vi "MacroEditor.vi"(2 "System":u16(ring) items=["Cusp", "Positron", "Musashi"], 3 "Save/Open Path":path=path "C:/CuspControl/Cusp/1_Macros/Antiprotons/Reservoir/Test1/scoop.mac", 4 "Sub-vi'd (open)":bool=TRUE) -> (1 "Saved at least once":bool=TRUE)   [LabVIEW 2018]
uses:
  MacroEditor Files/Instructions.ctl
  Executor Files/RT/Instruction.ctl
  Executor Files/VariableScan_Cluster.ctl
  MacroEditor Files/MacroSaveCluster.ctl
panel:
  in  "Tab Control":enum32{"Main", "Stored", "Basher"}(tab)
  in  "Instructions":T1=[{"Duration"=0.1, "Comment"="wait", "Steps"=1, "Edit Potential"=FALSE, "Output Bits"=[FALSE, FALSE, FALSE, FALSE, FALSE, FALSE, FALSE, FALSE, FALSE, FALSE, FALSE, FALSE, FALSE, FALSE, FALSE, FALSE, FALSE, FALSE, FALSE, FALSE, FALSE, FALSE, FALSE, FALSE, FALSE, FALSE, FALSE, FALSE, FALSE, FALSE, FALSE, FALSE, FALSE, FALSE, FALSE, FALSE, FALSE, FALSE], "Macro Path"=path "", "Potentials"=[-100.0, 0.0, -14.0, 0.0, 0.0, 0.0, -100.0, 0.0, 0.0, 0.0, 0.0, 0.0, 0.0, 0.0, 0.0, 0.0], "Inherit?"=FALSE}, {"Duration"=0.1, "Comment"="pbar to u8u9\nrw off", "Steps"=100, "Edit Potential"=FALSE, "Output Bits"=[FALSE, FALSE, FALSE, FALSE, FALSE, FALSE, FALSE, FALSE, FALSE, FALSE, FALSE, FALSE, FALSE, FALSE, FALSE, FALSE, FALSE, FALSE, FALSE, FALSE, FALSE, FALSE, FALSE, FALSE, FALSE, FALSE, FALSE, FALSE, FALSE, FALSE, FALSE, FALSE, FALSE, FALSE, FALSE, FALSE, FALSE, FALSE], "Macro Path"=path "", "Potentials"=[-100.0, 0.0, 0.0, 0.0, 20.0, 20.0, -100.0, 0.0, 0.0, 0.0, 0.0, 0.0, 0.0, 0.0, 0.0, 0.0], "Inherit?"=FALSE}, {"Duration"=0.1, "Comment"="match level", "Steps"=100, "Edit Potential"=FALSE, "Output Bits"=[FALSE, FALSE, FALSE, FALSE, FALSE, FALSE, FALSE, FALSE, FALSE, FALSE, FALSE, FALSE, FALSE, FALSE, FALSE, FALSE, FALSE, FALSE, FALSE, FALSE, FALSE, FALSE, FALSE, FALSE, FALSE, FALSE, FALSE, FALSE, FALSE, FALSE, FALSE, FALSE, FALSE, FALSE, FALSE, FALSE, FALSE, FALSE], "Macro Path"=path "", "Potentials"=[-100.0, 0.0, 0.0, 0.0, 1.93, 1.93, -100.0, 0.0, 0.0, 0.0, 0.0, 0.0, 0.0, 0.0, 0.0, 0.0], "Inherit?"=FALSE}, {"Duration"=0.1, "Comment"="scoop", "Steps"=100, "Edit Potential"=FALSE, "Output Bits"=[FALSE, FALSE, FALSE, FALSE, FALSE, FALSE, FALSE, FALSE, FALSE, FALSE, FALSE, FALSE, FALSE, FALSE, FALSE, FALSE, FALSE, FALSE, FALSE, FALSE, FALSE, FALSE, FALSE, FALSE, FALSE, FALSE, FALSE, FALSE, FALSE, FALSE, FALSE, FALSE, FALSE, FALSE, FALSE, FALSE, FALSE, FALSE], "Macro Path"=path "", "Potentials"=[-100.0, 80.0, -50.0, 0.0, 1.93, 1.93, -100.0, 0.0, 0.0, 0.0, 0.0, 0.0, 0.0, 0.0, 0.0, 0.0], "Inherit?"=FALSE}, {"Duration"=0.1, "Comment"="move\n12: u13 relay", "Steps"=100, "Edit Potential"=FALSE, "Output Bits"=[FALSE, FALSE, FALSE, FALSE, FALSE, FALSE, FALSE, FALSE, FALSE, FALSE, FALSE, FALSE, TRUE, FALSE, FALSE, FALSE, FALSE, FALSE, FALSE, FALSE, FALSE, FALSE, FALSE, FALSE, FALSE, FALSE, FALSE, FALSE, FALSE, FALSE, FALSE, FALSE, FALSE, FALSE, FALSE, FALSE, FALSE, FALSE], "Macro Path"=path "", "Potentials"=[-100.0, 70.0, -110.0, 0.0, 20.0, 20.0, -100.0, 0.0, 0.0, 0.0, 0.0, 0.0, 0.0, 0.0, 0.0, 0.0], "Inherit?"=FALSE}, {"Duration"=0.1, "Comment"="move\n", "Steps"=100, "Edit Potential"=FALSE, "Output Bits"=[FALSE, FALSE, FALSE, FALSE, FALSE, FALSE, FALSE, FALSE, FALSE, FALSE, FALSE, FALSE, TRUE, FALSE, FALSE, FALSE, FALSE, FALSE, FALSE, FALSE, FALSE, FALSE, FALSE, FALSE, FALSE, FALSE, FALSE, FALSE, FALSE, FALSE, FALSE, FALSE, FALSE, FALSE, FALSE, FALSE, FALSE, FALSE], "Macro Path"=path "", "Potentials"=[-100.0, -95.0, -110.0, 0.0, 20.0, 20.0, -100.0, 0.0, 0.0, 0.0, 0.0, 0.0, 0.0, 0.0, 0.0, 0.0], "Inherit?"=FALSE}, {"Duration"=0.005, "Comment"="01: ekick", "Steps"=1, "Edit Potential"=FALSE, "Output Bits"=[FALSE, TRUE, FALSE, FALSE, FALSE, FALSE, FALSE, FALSE, FALSE, FALSE, FALSE, FALSE, TRUE, FALSE, FALSE, FALSE, FALSE, FALSE, FALSE, FALSE, FALSE, FALSE, FALSE, FALSE, FALSE, FALSE, FALSE, FALSE, FALSE, FALSE, FALSE, FALSE, FALSE, FALSE, FALSE, FALSE, FALSE, FALSE], "Macro Path"=path "", "Potentials"=[-100.0, -95.0, -110.0, 0.0, 20.0, 20.0, -100.0, 0.0, 0.0, 0.0, 0.0, 0.0, 0.0, 0.0, 0.0, 0.0], "Inherit?"=TRUE}, {"Duration"=0.005, "Comment"="dump\n00: daq trig\n23: hodo trig", "Steps"=1, "Edit Potential"=FALSE, "Output Bits"=[TRUE, FALSE, FALSE, FALSE, FALSE, FALSE, FALSE, FALSE, FALSE, FALSE, FALSE, FALSE, TRUE, FALSE, FALSE, FALSE, FALSE, FALSE, FALSE, FALSE, FALSE, FALSE, FALSE, TRUE, FALSE, FALSE, FALSE, FALSE, FALSE, FALSE, FALSE, FALSE, FALSE, FALSE, FALSE, FALSE, FALSE, FALSE], "Macro Path"=path "", "Potentials"=[-100.0, -130.0, -110.0, 0.0, 20.0, 20.0, -100.0, 0.0, 0.0, 0.0, 0.0, 0.0, 0.0, 0.0, 0.0, 0.0], "Inherit?"=FALSE}, {"Duration"=0.01, "Comment"="recover", "Steps"=100, "Edit Potential"=FALSE, "Output Bits"=[FALSE, FALSE, FALSE, FALSE, FALSE, FALSE, FALSE, FALSE, FALSE, FALSE, FALSE, FALSE, FALSE, FALSE, FALSE, FALSE, FALSE, FALSE, FALSE, FALSE, FALSE, FALSE, FALSE, FALSE, FALSE, FALSE, FALSE, FALSE, FALSE, FALSE, FALSE, FALSE, FALSE, FALSE, FALSE, FALSE, FALSE, FALSE], "Macro Path"=path "", "Potentials"=[-100.0, 0.0, -14.0, 0.0, 20.0, 20.0, -100.0, 0.0, 0.0, 0.0, 0.0, 0.0, 0.0, 0.0, 0.0, 0.0], "Inherit?"=FALSE}, {"Duration"=0.1, "Comment"="back to rw well", "Steps"=100, "Edit Potential"=FALSE, "Output Bits"=[FALSE, FALSE, FALSE, FALSE, FALSE, FALSE, FALSE, FALSE, FALSE, FALSE, FALSE, FALSE, FALSE, FALSE, FALSE, FALSE, FALSE, FALSE, FALSE, FALSE, FALSE, FALSE, FALSE, FALSE, FALSE, FALSE, FALSE, FALSE, FALSE, FALSE, FALSE, FALSE, FALSE, FALSE, FALSE, FALSE, FALSE, FALSE], "Macro Path"=path "", "Potentials"=[-100.0, 0.0, -14.0, 0.0, 0.0, 0.0, -100.0, 0.0, 0.0, 0.0, 0.0, 0.0, 0.0, 0.0, 0.0, 0.0], "Inherit?"=FALSE}] {"Steps" min=1 max=100000 step=1; "Duration" min=0.001 step=0.001 format="%_6p"}
  in  "stop":bool
  in  "Save":bool
  in  "Open":bool
  in  "New":bool
  in  "Macro Description":string="start and end in pbar rw well\ne+ stay in u7 = -100 V"
  in  "Copy Inst.":bool
  out "Changes":bool[][](array[boolean])=[[TRUE, TRUE], [FALSE, TRUE], [FALSE, TRUE], [FALSE, TRUE], [TRUE, TRUE], [FALSE, TRUE], [TRUE, FALSE], [TRUE, TRUE], [TRUE, TRUE], [FALSE, TRUE]]
  out "message":string="Input Bit Assignments\n-------------------------\n01 pbar sync\n02 e+ sync\n\nOutput Bit Assignments\n-------------------------\n00 DAQ trigger\n01 HV pulser(s) trigger\n02 \n03 MCP select\n04 MCP in\n05 MCP out\n06 e- source select\n07 e- source insert\n08 e- source remove\n09 pulsed coil enable\n10 Brescia trigger\n11 Relays - u10\n12 AC bypass relay - u13\n13 Entrance GV open\n14 Entrance GV close\n15 bk4054b gate - u5\n16 bk4054b gate - u10\n17 Higaki B-C fire\n18 Higaki A fire\n19 Tajima fire\n20 Tanaka fire\n21 Exit GV open\n22 Exit GV close\n23 BGO gate\n24 bk4054b gate - u4"
  out "# Instructions":i32=10
  out "Total time (s)":dbl=0.738 format="%_4p"
  in  "Analog buffer (2 ms)":dbl=0.002 format="%#_3p"
  in  "Path tag":string="t"
  in  "Variable Cluster":T3={"Values"=[2.78, 1.795, 0.81, -0.17499999999999982, -1.16], "Action"=1, "Inst."=2, "# Elements"=5, "Next Element"=0, "First Val"=2.78, "Final Val"=-1.16, "Update Array"=FALSE, "Description"="", "Variable Type"=1, "Scan Now"=FALSE, "# Act/Inst."=2, "Electrodes_range"=[], "Parameter Name"="RW&f_start (Hz)", "# Passes"=1} {"Variable Type" items=["Duration (s)", "Voltage (V)", "Parameter", "Repetitions"]; "Final Val" format="%_6p"; "First Val" format="%_6p"; "Values" format="%_6p"}
  out "Edit #":i32=-1
  # "0        2       4       6        8      10     12     14     16     18      20    22     24     26     28     30     32     34     36"
  # "Digital and Analog 'Changes' is only updated when you Save"
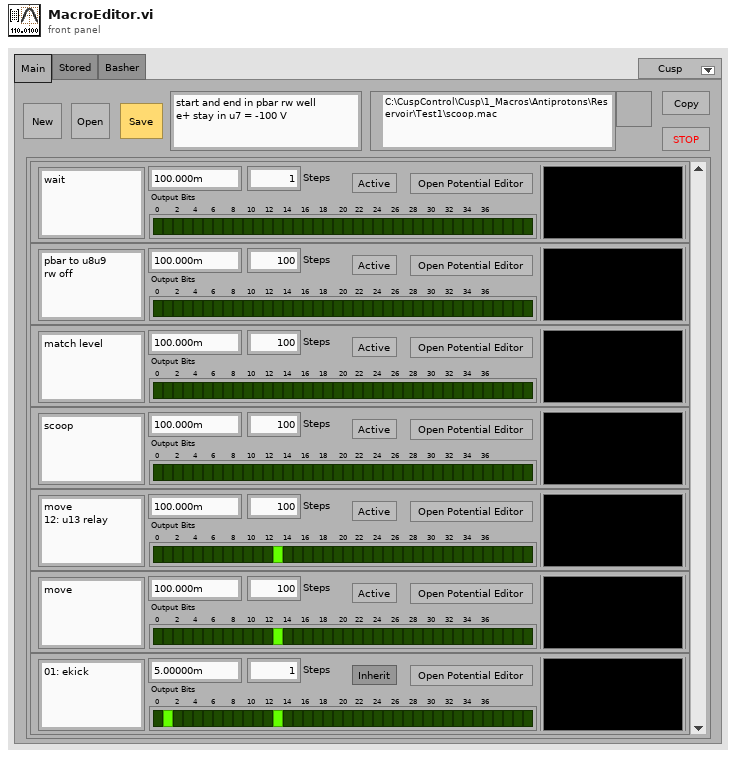
[diagram p1: front panel]
types:
  T1 = typedef "Instructions.ctl" = T2[]
  T2 = typedef "Instruction.ctl" = cluster{"Duration":dbl, "Comment":string, "Steps":i32, "Edit Potential":bool, "Output Bits":bool[], "Macro Path":path, "Potentials":dbl[], "Inherit?":bool}
  T3 = typedef "VariableScan_Cluster.ctl" = cluster{"Values":dbl[], "Action":i32, "Inst.":i32, "# Elements":i32, "Next Element":i32, "First Val":dbl, "Final Val":dbl, "Update Array":bool, "Description":string, "Variable Type":u16, "Scan Now":bool, "# Act/Inst.":i32, "Electrodes_range":i32[], "Parameter Name":string, "# Passes":i32}
  T4 = typedef "MacroSaveCluster.ctl" = cluster{"Instructions":T1, "Changes":bool[][], "Macro Description":string, "Total Time (s)":dbl, "Samples per sec":dbl}
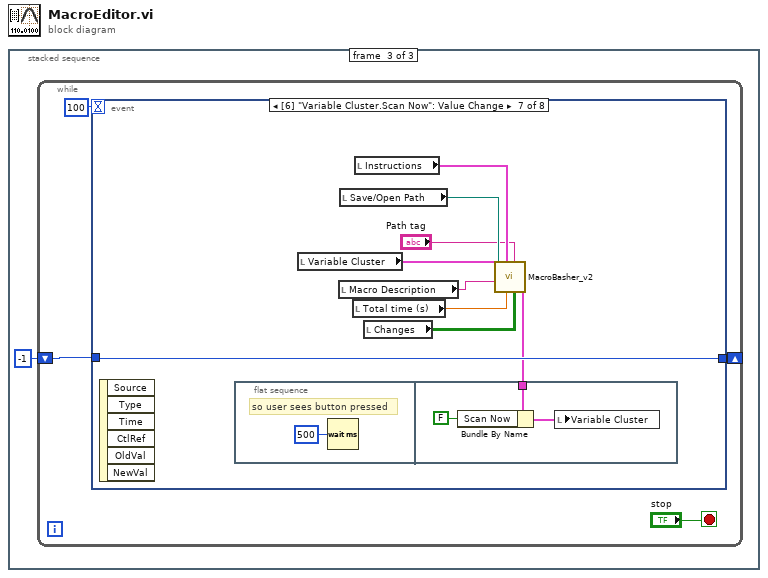
[diagram p0: block diagram]
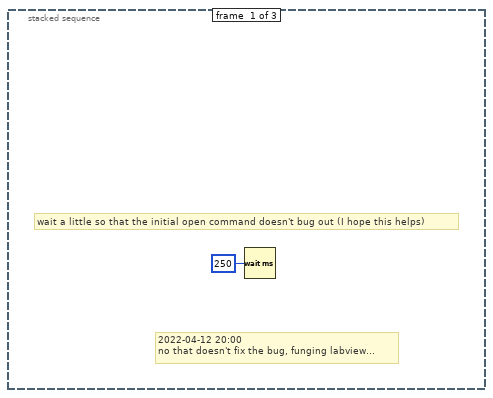
[diagram p2: hidden frame]
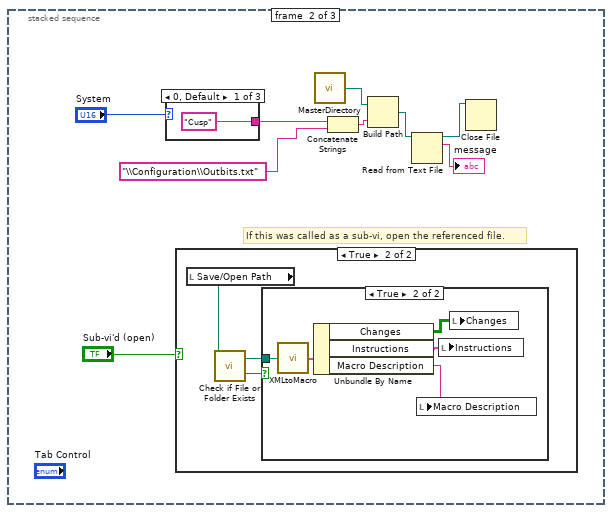
[diagram p3: hidden frame]
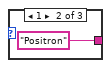
[diagram p4: hidden frame]
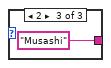
[diagram p5: hidden frame]
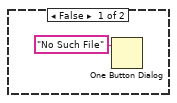
[diagram p7: hidden frame]
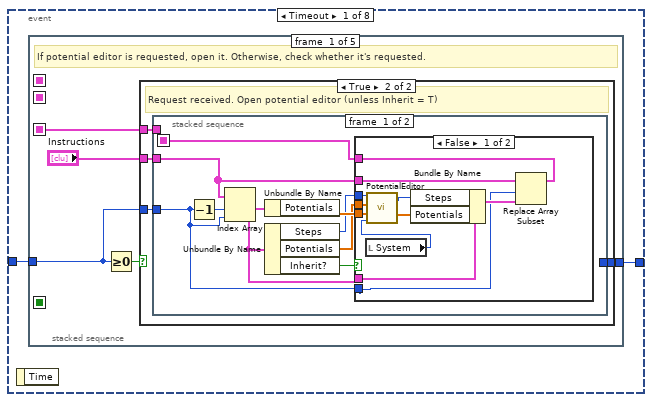
[diagram p8: hidden frame]
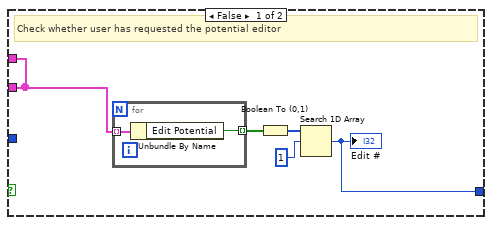
[diagram p9: hidden frame]
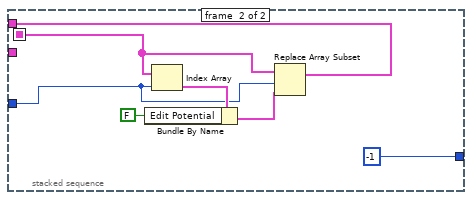
[diagram p11: hidden frame]
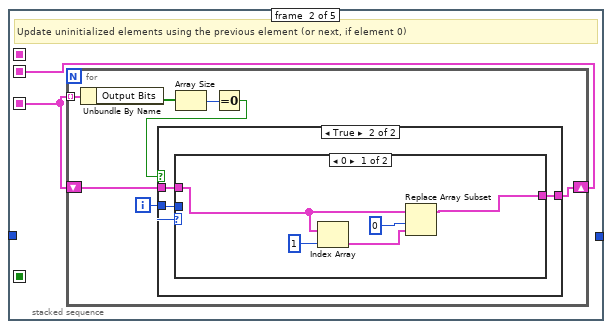
[diagram p12: hidden frame]
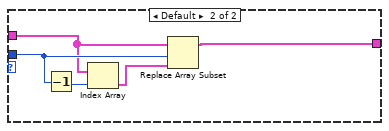
[diagram p14: hidden frame]
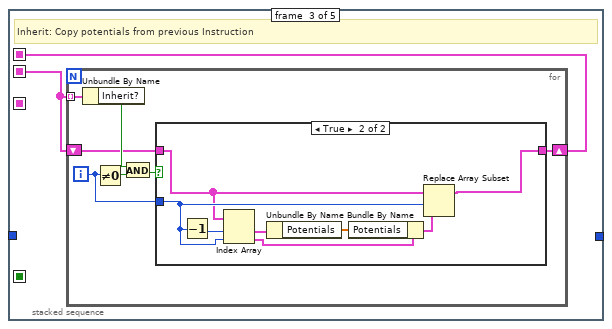
[diagram p15: hidden frame]
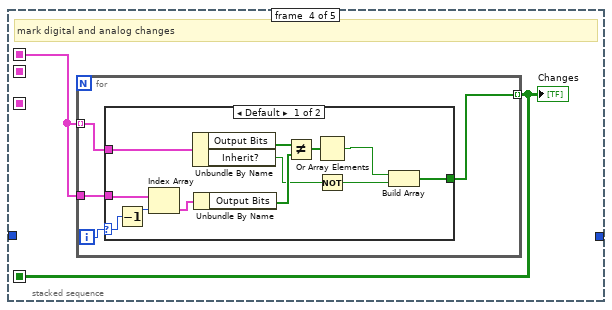
[diagram p17: hidden frame]
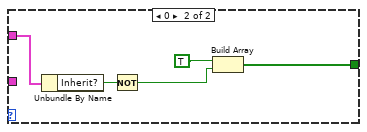
[diagram p18: hidden frame]
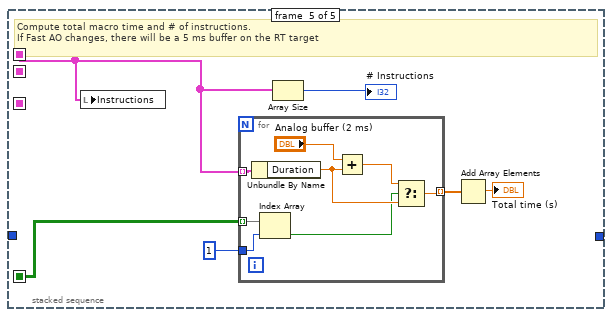
[diagram p19: hidden frame]
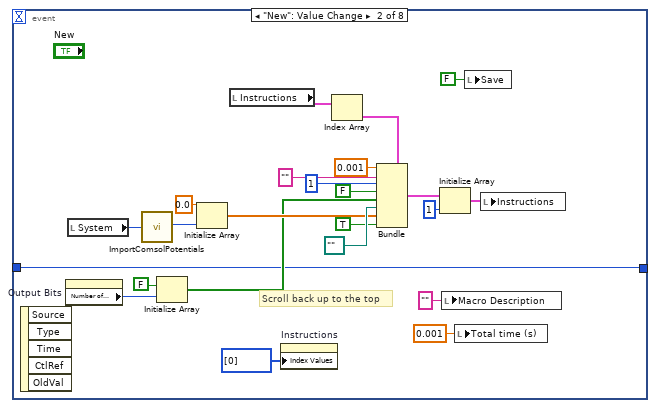
[diagram p20: hidden frame]
diagram:
  n1 = stacked-sequence {
    frame #0 {
      # "2022-04-12 20:00\nno that doesn't fix the bug, funging labview..."
      # "wait a little so that the initial open command doesn't bug out (I hope this helps)"
      n2 = Wait (ms)(milliseconds to wait=u32 250) -> ()  [unwired: 1 out]
    }
    frame #1 {
      # "If this was called as a sub-vi, open the referenced file."
      n3 = case shown="0, Default" "System" {
        tunnel: ["Cusp" ("string") "Positron" ("string") "Musashi" ("string")] -> w9
        frame 0, Default {
        }
        frame 1 {
        }
        frame 2 {
        }
      }
      n4 = case shown="True" "Sub-vi'd (open)" {
        frame False {
        }
        frame True {
          n5 = local read "Save/Open Path"() -> (w14:path)
          n6 = call <vilib>:"Check if File or Folder Exists.vi"("path"=w14) -> ("file or folder exists?"=w16:bool, "dup path"=w15:path)  [unwired: 8 in, 1 out]
          n7 = case shown="True" w16 {
            tunnel: w15 -> [_ w22]
            frame False {
              n8 = One Button Dialog(message="No Such File") -> ()  [unwired: 1 in, 1 out]
            }
            frame True {
              n9 = call "XMLtoMacro.vi"("XML File Path"=w22) -> ("MacroSaveCluster"=w21:T4)
              n10 = Unbundle By Name(w21) -> ("Changes"=w19:bool[][], "Instructions"=w18:T1, "Macro Description"=w20:string)
              n11 = local write "Macro Description"(w20) -> ()
              n12 = local write "Instructions"(w18) -> ()
              n13 = local write "Changes"(w19) -> ()
            }
          }
        }
      }
      n14 = call "MasterDirectory.vi"() -> ("Master Directory"=w5:path)
      n15 = Concatenate Strings(w9, "\\Configuration\\Outbits.txt" ("string")) -> (w4:string)
      n16 = Build Path(base path=w5, name or relative path=w4) -> (appended path=w3:path)
      n17 = Read from Text File(file (use dialog)=w3) -> (refnum out=w6:refnum<file>, text=→"message":string)  [unwired: 3 in, 2 out]
      n18 = Close File(refnum=w6) -> ()  [unwired: 1 in, 2 out]
    }
    frame #2 {
      n19 = while {
        shift-right: [w24] -> _
        shift-left: -1 ("Edit #") -> [w25]
        stop <- "stop" stop-if-true
        n20 = event shown="[6] \"Variable Cluster.Scan Now\": Value Change" {
          selector: _ -> [_ _ _ _ _ _ _ _]
          dyn-events: _ -> [_ _ _ _ _ _ _ _]
          timeout: 100 -> [_ _ _ _ _ _ _ _]
          tunnel: w25 -> [w29 w153 w176 w188 w199 w201 w213 w219]
          tunnel: [w28 w153 w176 w188 w199 w201 w213 w219] -> w24
          event Timeout {
            n21 = event-data() -> ()  [unwired: 1 in, 1 out]
            n22 = stacked-sequence {
              seq-local: [w32 _ _ _ _] -> [_ w76 _ _ _]
              seq-local: [_ w75 _ _ _] -> [_ _ w99 _ _]
              seq-local: [_ _ w98 _ _] -> [_ _ _ w117 w139]
              seq-local: [_ _ _ w116 _] -> [_ _ _ _ w140]
              tunnel: w29 -> [w31 _ _ _ _]
              tunnel: [w30 _ _ _ _] -> w28
              frame #0 {
                # "If potential editor is requested, open it. Otherwise, check whether it's requested."
                n23 = Greater Or Equal To 0?(x=w31) -> (x >= 0?=w34:bool)
                n24 = case shown="True" w34 {
                  tunnel: w31 -> [_ w45]
                  tunnel: "Instructions" -> [w36 w44]
                  tunnel: [w36 w43] -> w32
                  tunnel: [w35 w42] -> w30
                  frame False {
                    # "Check whether user has requested the potential editor"
                    n25 = for {
                      tunnel: w36 -> [w41] mode=indexing
                      tunnel: [w40] -> w37 mode=indexing
                      n26 = Unbundle By Name(w41) -> ("Edit Potential"=w40:bool)
                    }
                    n27 = Boolean To (0,1)(Boolean=w37) -> (0, 1=w39:i16[])
                    n28 = Search 1D Array(1D array=w39, element=1) -> (index of element=w35:i32)  [unwired: 1 in]
                    "Edit #" <- w35
                  }
                  frame True {
                    # "Request received. Open potential editor (unless Inherit = T)"
                    n29 = stacked-sequence {
                      seq-local: [w47 _] -> [_ w70]
                      tunnel: w45 -> [w46 w72]
                      tunnel: w44 -> [w48 _]
                      tunnel: [_ w69] -> w43
                      tunnel: [_ -1 ("Edit #")] -> w42
                      frame #0 {
                        n30 = Decrement(x=w46) -> (x-1=w55:i32)
                        n31 = Index Array(array=w48, index #1=w55, index #2=w46) -> (element #1=w54:T2, element #2=w50:T2)
                        n32 = Unbundle By Name(w54) -> ("Potentials"=w53:dbl[])
                        n33 = Unbundle By Name(w50) -> ("Steps"=w51:i32, "Potentials"=w52:dbl[], "Inherit?"=w49:bool)
                        n34 = case shown="False" w49 {
                          tunnel: w53 -> [w66 _]
                          tunnel: w52 -> [w65 _]
                          tunnel: w51 -> [w64 _]
                          tunnel: w50 -> [w63 _]
                          tunnel: w48 -> [w59 w67]
                          tunnel: [w57 w67] -> w47
                          tunnel: w46 -> [w56 _]
                          frame False {
                            n35 = local read "System"() -> (w58:u16)
                            n36 = call "PotentialEditor.vi"("System"=w58, "Previous Excitations in"=w66, "Requested"=w65, "Steps"=w64) -> ("Excitations Out"=w62:dbl[], "Steps Out"=w61:i32)
                            n37 = Bundle By Name(cluster=w63, "Steps"=w61, "Potentials"=w62) -> (w60:T2)
                            n38 = Replace Array Subset(array=w59, new element=w60, index=w56) -> (w57:T1)
                          }
                          frame True {
                          }
                        }
                      }
                      frame #1 {
                        n39 = Index Array(array=w70, index=w72) -> (element=w74:T2)
                        n40 = Bundle By Name(cluster=w74, "Edit Potential"=FALSE) -> (w71:T2)
                        n41 = Replace Array Subset(array=w70, new element=w71, index=w72) -> (w69:T1)
                      }
                    }
                  }
                }
              }
              frame #1 {
                # "Update uninitialized elements using the previous element (or next, if element 0)"
                n42 = for {
                  tunnel: w76 -> [w83] mode=indexing
                  shift-right: [w77] -> w75
                  shift-left: w76 -> [w78]
                  i -> [w80]
                  n43 = Unbundle By Name(w83) -> ("Output Bits"=w82:bool[])
                  n44 = Array Size(array=w82) -> (size(s)=w81:i32)
                  n45 = Equal To 0?(x=w81) -> (x = 0?=w79:bool)
                  n46 = case shown="True" w79 {
                    tunnel: w80 -> [_ w87]
                    tunnel: w78 -> [w84 w86]
                    tunnel: [w84 w85] -> w77
                    frame False {
                    }
                    frame True {
                      n47 = case shown="0" w87 {
                        tunnel: w87 -> [_ w96]
                        tunnel: w86 -> [w89 w94]
                        tunnel: [w88 w93] -> w85
                        frame 0 {
                          n48 = Index Array(array=w89, index=1) -> (element=w90:T2)
                          n49 = Replace Array Subset(array=w89, new element=w90, index=0) -> (w88:T1)
                        }
                        frame Default {
                          n50 = Decrement(x=w96) -> (x-1=w97:i32)
                          n51 = Index Array(array=w94, index=w97) -> (element=w95:T2)
                          n52 = Replace Array Subset(array=w94, new element=w95, index=w96) -> (w93:T1)
                        }
                      }
                    }
                  }
                }
              }
              frame #2 {
                # "Inherit: Copy potentials from previous Instruction"
                n53 = for {
                  tunnel: w99 -> [w106] mode=indexing
                  shift-right: [w100] -> w98
                  shift-left: w99 -> [w101]
                  i -> [w103]
                  n54 = Unbundle By Name(w106) -> ("Inherit?"=w104:bool)
                  n55 = Not Equal To 0?(x=w103) -> (x != 0?=w102:bool)
                  n56 = And(x=w104, y=w102) -> (x .and. y?=w105:bool)
                  n57 = case shown="True" w105 {
                    tunnel: w103 -> [_ w113]
                    tunnel: w101 -> [w107 w109]
                    tunnel: [w107 w108] -> w100
                    frame False {
                    }
                    frame True {
                      n58 = Decrement(x=w113) -> (x-1=w115:i32)
                      n59 = Index Array(array=w109, index #1=w115, index #2=w113) -> (element #1=w114:T2, element #2=w112:T2)
                      n60 = Unbundle By Name(w114) -> ("Potentials"=w111:dbl[])
                      n61 = Bundle By Name(cluster=w112, "Potentials"=w111) -> (w110:T2)
                      n62 = Replace Array Subset(array=w109, new element=w110, index=w113) -> (w108:T1)
                    }
                  }
                }
              }
              frame #3 {
                # "mark digital and analog changes"
                n63 = for {
                  tunnel: w117 -> [w120] mode=indexing
                  tunnel: [w118] -> w116 mode=indexing
                  tunnel: w117 -> [w119]
                  i -> [w121]
                  n64 = case shown="Default" w121 {
                    selector: w121 -> [w131 _]
                    tunnel: [w124 w137] -> w118
                    tunnel: w120 -> [w130 w136]
                    tunnel: w119 -> [w133 _]
                    frame Default {
                      n65 = Decrement(x=w131) -> (x-1=w132:i32)
                      n66 = Index Array(array=w133, index=w132) -> (element=w129:T2)
                      n67 = Unbundle By Name(w130) -> ("Output Bits"=w128:bool[], "Inherit?"=w123:bool)
                      n68 = Unbundle By Name(w129) -> ("Output Bits"=w127:bool[])
                      n69 = Not Equal?(x=w128, y=w127) -> (x != y?=w126:bool[])
                      n70 = Or Array Elements(Boolean array=w126) -> (logical OR=w125:bool)
                      n71 = Not(x=w123) -> (.not. x?=w122:bool)
                      n72 = Build Array(w125, w122) -> (w124:bool[])
                    }
                    frame 0 {
                      n73 = Unbundle By Name(w136) -> ("Inherit?"=w135:bool)
                      n74 = Not(x=w135) -> (.not. x?=w134:bool)
                      n75 = Build Array(TRUE, w134) -> (w137:bool[])
                    }
                  }
                }
                "Changes" <- w116
              }
              frame #4 {
                # "Compute total macro time and # of instructions.\nIf Fast AO changes, there will be a 5 ms buffer on the RT target"
                n76 = local write "Instructions"(w139) -> ()
                n77 = for {
                  tunnel: w139 -> [w152] mode=indexing
                  tunnel: [w150] -> w144 mode=indexing
                  tunnel: w140 -> [w147] mode=indexing
                  tunnel: 1 ("index") -> [w146]
                  n78 = Unbundle By Name(w152) -> ("Duration"=w148:dbl)
                  n79 = Index Array(array=w147, index=w146) -> (element=w145:bool)
                  n80 = Add(x="Analog buffer (2 ms)", y=w148) -> (x+y=w149:dbl)
                  n81 = Select(t=w149, s=w145, f=w148) -> (s? t:f=w150:dbl)
                }
                n82 = Array Size(array=w139) -> (size(s)=→"# Instructions":i32)
                n83 = Add Array Elements(numeric array=w144) -> (sum=→"Total time (s)":dbl)
              }
            }
          }
          event "New": Value Change {
            # "Scroll back up to the top"
            n84 = event-data() -> ()  [unwired: 1 in, 5 out]
            n85 = property on="Output Bits" class="Arr (strict)"() -> ("Number of Columns"=w156:u32)  [unwired: 2 in, 2 out]
            n86 = local read "System"() -> (w161:u16)
            n87 = call "ImportComsolPotentials.vi"("System"=w161) -> ("# electrodes"=w170:i32)  [unwired: 2 out]
            n88 = Initialize Array(FALSE, w156) -> (w155:bool[])
            n89 = Initialize Array(0.0, w170) -> (w157:dbl[])
            n90 = local read "Instructions"() -> (w166:T1)
            n91 = property on="Instructions" class="Arr"("Index Values"=u32[] [0]) -> ()  [unwired: 2 in, 2 out]
            n92 = Index Array(array=w166) -> (element=w165:T2)  [unwired: 1 in]
            n93 = Bundle(cluster=w165, "Duration"=0.001, "Comment"="", "Steps"=1, "Edit Potential"=FALSE, "Output Bits"=w155, "Macro Path"=path "", "Potentials"=w157, "Inherit?"=TRUE ("Edit Potential")) -> (w175:T2)
            n94 = Initialize Array(w175, 1 ("dimension size")) -> (w173:T2[])
            n95 = local write "Macro Description"("" ("Macro Description")) -> ()
            n96 = local write "Total time (s)"(0.001 ("Total time (s)")) -> ()
            n97 = local write "Save"(FALSE ("Save")) -> ()
            n98 = local write "Instructions"(w173) -> ()
          }
          event "Save": Value Change {
            n99 = event-data() -> ()  [unwired: 1 in, 3 out]
            n100 = case shown="True" "Save" {
              tunnel: "Save/Open Path" -> [_ w187]
              frame False {
              }
              frame True {
                w181 = 1.0  # Samples per sec (legacy)
                n101 = local read "Total time (s)"() -> (w184:dbl)
                n102 = local read "Changes"() -> (w180:bool[][])
                n103 = local read "Instructions"() -> (w186:T1)
                n104 = Bundle(cluster=T4 {"Instructions"=[], "Changes"=[], "Macro Description"="", "Total Time (s)"=0.0, "Samples per sec"=0.0} ("output cluster"), "Instructions"=w186, "Changes"=w180, "Macro Description"="Macro Description", "Total Time (s)"=w184, "Samples per sec"=w181) -> (w183:T4)
                n105 = call "MacrotoXML.vi"("MacroSaveCluster"=w183, "XML File Path"=w187) -> ()  [unwired: 1 in]
              }
            }
            "Saved at least once" <- TRUE ("Saved at least once")
          }
          event "Open": Value Change {
            # "Scroll back up to the top"
            n106 = event-data() -> ()  [unwired: 1 in, 3 out]
            n107 = local read "Save/Open Path"() -> (w192:path)
            n108 = call <vilib>:"Check if File or Folder Exists.vi"("path"=w192) -> ("file or folder exists?"=w191:bool, "dup path"=w190:path)  [unwired: 8 in, 1 out]
            n109 = case shown="True" w191 {
              tunnel: w190 -> [_ w198]
              frame False {
                n110 = One Button Dialog(message="No Such File") -> ()  [unwired: 1 in, 1 out]
              }
              frame True {
                n111 = call "XMLtoMacro.vi"("XML File Path"=w198) -> ("MacroSaveCluster"=w195:T4)
                n112 = Unbundle By Name(w195) -> ("Instructions"=w197:T1, "Macro Description"=w196:string, "Changes"=w194:bool[][])
                n113 = local write "Instructions"(w197) -> ()
                n114 = local write "Macro Description"(w196) -> ()
                n115 = local write "Changes"(w194) -> ()
              }
            }
            n116 = property on="Instructions" class="Arr"("Index Values"=u32[] [0]) -> ()  [unwired: 2 in, 2 out]
          }
          event "Macro Description": Mouse Down {
            # "(stale)"
            n117 = event-data() -> ()  [unwired: 1 in, 5 out]
            n118 = local write "Save"(FALSE ("Save")) -> ()
          }
          event "Copy Inst.": Value Change {
            # "(stale)"
            n119 = event-data() -> ()  [unwired: 1 in, 6 out]
            n120 = local write "Save"(FALSE ("Save")) -> ()
            n121 = local read "Instructions"() -> (w205:T1)
            n122 = call "CopyInstruction.vi"() -> ("Instruction to copy"=w203:T2, "Insert Index"=w204:u32)  [unwired: 1 in]
            n123 = Insert Into Array(array=w205, index=w204, new element=w203) -> (w202:T1)
            n124 = local write "Instructions"(w202) -> ()
          }
          event Value Change {
            n125 = event-data() -> ()  [unwired: 1 in, 6 out]
            n126 = flat-sequence {
              tunnel: w207 -> [w218]
              frame #0 {
                # "so user sees button pressed"
                n127 = Wait (ms)(milliseconds to wait=u32 500) -> ()  [unwired: 1 out]
              }
              frame #1 {
                n128 = Bundle By Name(cluster=w218, "Scan Now"=FALSE) -> (w216:T3)
                n129 = local write "Variable Cluster"(w216) -> ()
              }
            }
            n130 = local read "Variable Cluster"() -> (w207:T3)
            n131 = local read "Macro Description"() -> (w212:string)
            n132 = local read "Save/Open Path"() -> (w209:path)
            n133 = local read "Total time (s)"() -> (w210:dbl)
            n134 = local read "Instructions"() -> (w214:T1)
            n135 = local read "Changes"() -> (w211:bool[][])
            n136 = call "MacroBasher_v2.vi"("Changes"=w211, "Path tag"="Path tag", "Total time (s)"=w210, "Instructions"=w214, "Macro Description"=w212, "Variable Cluster"=w207, "Save/Open Path"=w209) -> ()  [unwired: 5 in]
          }
          event Value Change {
            n137 = event-data() -> ()  [unwired: 1 in, 6 out]
            n138 = Unbundle By Name("Variable Cluster") -> ("First Val"=w223:dbl, "Final Val"=w224:dbl, "# Elements"=w225:i32, "# Passes"=w226:i32)
            n139 = call "GenerateInterleavedList.vi"("# passes"=w226, "# points"=w225, "Stop"=w224, "Start"=w223) -> ("Array"=w227:dbl[])  [unwired: 2 in, 1 out]
            n140 = Bundle By Name(cluster="Variable Cluster", "Values"=w227, "Update Array"=FALSE) -> (w222:T3)
            n141 = local write "Variable Cluster"(w222) -> ()
          }
        }
      }
    }
  }
